vi "Get Specific Regexp.vi"(11 "key of line, of matrix, of section ('')":string) -> (0 "Any Section":string="(?ms)^\\h*#startsection\\h*::\\h*([^\\n]*)\\h*(?:\\n(.*)\\n|\\n)^\\h*#endsection\\h*::\\h*\\1\\h*$", 1 "Section":string="(?ms)^\\h*#startsection\\h*::\\h*([^\\n]*)\\h*(?:\\n(.*)\\n|\\n)^\\h*#endsection\\h*::\\h*\\1\\h*$", 2 "Matrix":string="(?ms)^\\h*#startsection\\h*::\\h*([^\\n]*)\\h*(?:\\n(.*)\\n|\\n)^\\h*#endsection\\h*::\\h*\\1\\h*$", 3 "Line":string="(?ms)^\\h*#startsection\\h*::\\h*([^\\n]*)\\h*(?:\\n(.*)\\n|\\n)^\\h*#endsection\\h*::\\h*\\1\\h*$")   [LabVIEW 2020, in "infolib.lvlib"]
doc: "Returns regexps used in infostrings. This vi is to keep all regexps at one place for better review.\nThe key is used to generate specific regexps. The key is translated for special characters inside this vi."
uses:
  infolib.lvlib
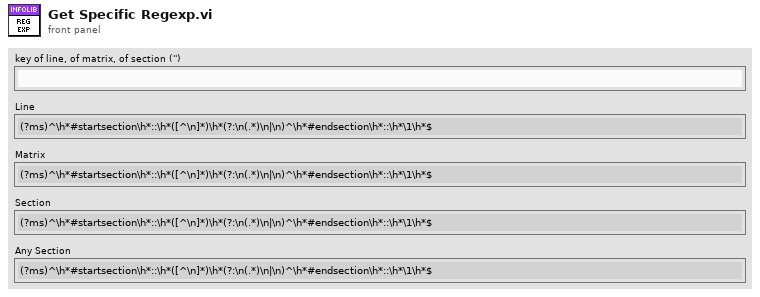
[diagram p1: front panel]
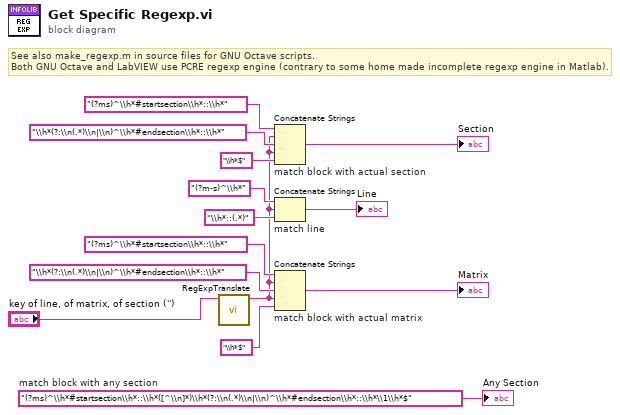
[diagram p0: block diagram]
diagram:
  w14 = "(?ms)^\\h*#startsection\\h*::\\h*([^\\n]*)\\h*(?:\\n(.*)\\n|\\n)^\\h*#endsection\\h*::\\h*\\1\\h*$"  # match block with any section
  # "See also make_regexp.m in source files for GNU Octave scripts.\nBoth GNU Octave and LabVIEW use PCRE regexp engine (contrary to some home made incomplete regexp engine in Matlab)."
  n1 = call "RegExpTranslate.vi"("string"="key of line, of matrix, of section ('')") -> ("regexp safe string"=w1:string)  [unwired: 10 in]
  n2 = Concatenate Strings "match block with actual section"("(?ms)^\\h*#startsection\\h*::\\h*" ("match block with actual section"), w1, "\\h*(?:\\n(.*)\\n|\\n)^\\h*#endsection\\h*::\\h*" ("match block with actual section"), w1, "\\h*$" ("match block with actual section")) -> (→"Section":string)
  n3 = Concatenate Strings "match line"("(?m-s)^\\h*" ("match block with actual section"), w1, "\\h*::(.*)" ("match block with actual section")) -> (→"Line":string)
  n4 = Concatenate Strings "match block with actual matrix"("(?ms)^\\h*#startsection\\h*::\\h*" ("match block with actual section"), w1, "\\h*(?:\\n(.*)\\n|\\n)^\\h*#endsection\\h*::\\h*" ("match block with actual section"), w1, "\\h*$" ("match block with actual section")) -> (→"Matrix":string)
  "Any Section" <- w14
